vi "VFP Network Set One Buffering Attr.vi"(8 "Ctrl Info":T2, 9 "Ctrl Ref":refnum<vi>, 10 "attribute name":string, 11 "attributes in":T1) -> (3 "attributes out":T1)   [LabVIEW 2016]
uses:
  <resource>/dialog/variable/SCT Attributes.ctl
  <resource>/dialog/variable/FeaturePacks/Network/VFP Network Control Info.ctl
  <resource>/dialog/variable/FeaturePacks/Utility/VFP Util Fetch String Control.vi
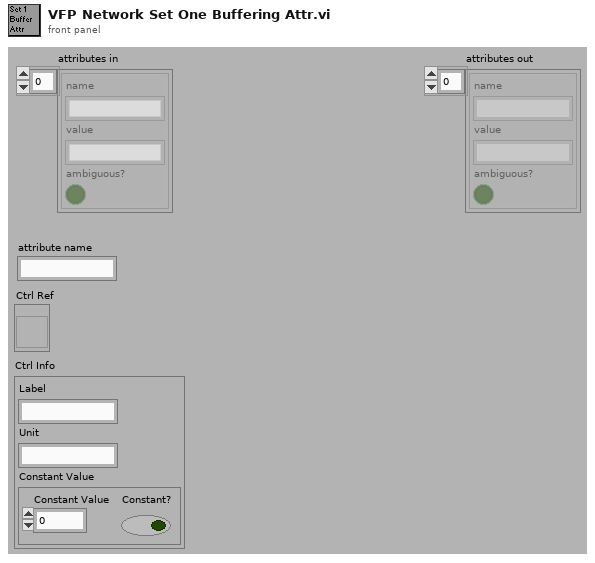
[diagram p1: front panel]
types:
  T1 = typedef "SCT Attributes.ctl" = cluster{"name":string, "value":string, "ambiguous?":bool}[]
  T2 = typedef "VFP Network Control Info.ctl" = cluster{"Label":string, "Unit":string, "Constant Value":cluster{"Constant Value":u32, "Constant?":bool}}
  T3 = cluster{"name":string, "value":string, "ambiguous?":bool}
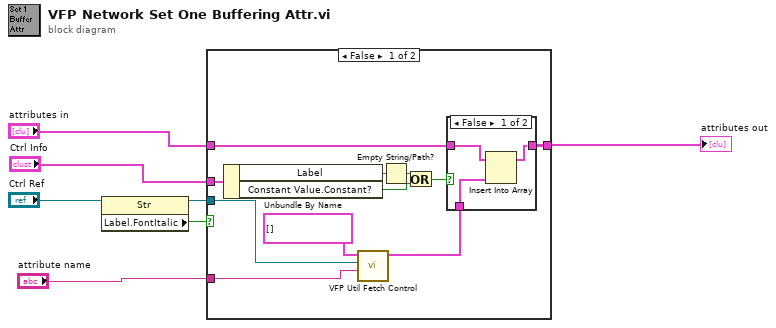
[diagram p0: block diagram]
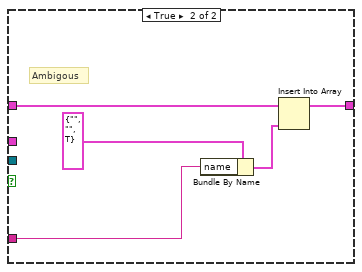
[diagram p3: hidden frame]
diagram:
  n1 = property class="Str"(reference="Ctrl Ref") -> (reference out=w5:refnum<vi>, "Label.FontItalic"=w2:bool)  [unwired: 1 in, 1 out]
  n2 = case shown="False" w2 {
    tunnel: "attributes in" -> [w11 w27]
    tunnel: [w10 w26] -> w7
    tunnel: "Ctrl Info" -> [w15 _]
    tunnel: w5 -> [w13 _]
    tunnel: "attribute name" -> [w12 w23]
    frame False {
      n3 = Unbundle By Name(w15) -> ("Label"=w16:string, "Constant Value.Constant?"=w17:bool)
      n4 = call-poly <resource>:"VFP Util Fetch Control.vi"("attribute name"=w12, "control"=w13, "attributes"=T1 []) -> ("attributes out"=w9:T1)  [unwired: 8 in]
      n5 = Empty String/Path?(string/path=w16) -> (empty?=w18:bool)
      n6 = Or(x=w18, y=w17) -> (x .or. y?=w8:bool)
      n7 = case shown="False" w8 {
        tunnel: w11 -> [w21 w22]
        tunnel: [w20 w22] -> w10
        tunnel: w9 -> [w19 _]
        frame False {
          n8 = Insert Into Array(array=w21, new element=w19) -> (w20:T1)  [unwired: 1 in]
        }
        frame True {
        }
      }
    }
    frame True {
      # "Ambigous"
      n9 = Bundle By Name(cluster=T3 {"name"="", "value"="", "ambiguous?"=TRUE} ("attribute"), "name"=w23) -> (w24:T3)
      n10 = Insert Into Array(array=w27, new element=w24) -> (w26:T1)  [unwired: 1 in]
    }
  }
  "attributes out" <- w7
